vi "Bind Control Caption.vi"(4 "Ignore Past Updates? (F)":bool, 8 "error in (no error)":errorcluster, 9 "Datum Name (\"\"=Use Control Label)":string, 10 "Control Refnum":refnum<vi>, 11 "IViewable in":refnum<class "IViewable.lvclass">) -> (0 "error out":errorcluster, 3 "IViewable out":refnum<class "IViewable.lvclass">)   [LabVIEW 2018, in "MVA Framework.lvlib" / "IViewable.lvlib" / "IViewable.lvclass"]
doc: "将控制终端（控件或指示器）的标题绑定到已发布的字符串。"
uses:
  IViewable.lvclass
  mva-core/Source/IMediator/SubscriptionRequest/SubscriptionRequest.lvclass
  mva-core/Source/IObserver/IObserver Messages/Subscribe Msg/Subscribe Msg.lvclass
  <vilib>/ActorFramework/Actor/Actor.lvclass
  mva-core/Source/IMediator/ISubscriptionPolicy/ISubscriptionPolicy.lvclass
  mva-core/Source/SubscriptionPolicy/ValueChangeSubscription/ValueChangeSubscription.lvclass
  composed-transport/Source/Concrete/TerminalCaptionBinding/TerminalCaptionBinding.lvclass
  C:/Program Files (x86)/National Instruments/LabVIEW 2020/vi.lib/ActorFramework/Actor/Actor.lvclass
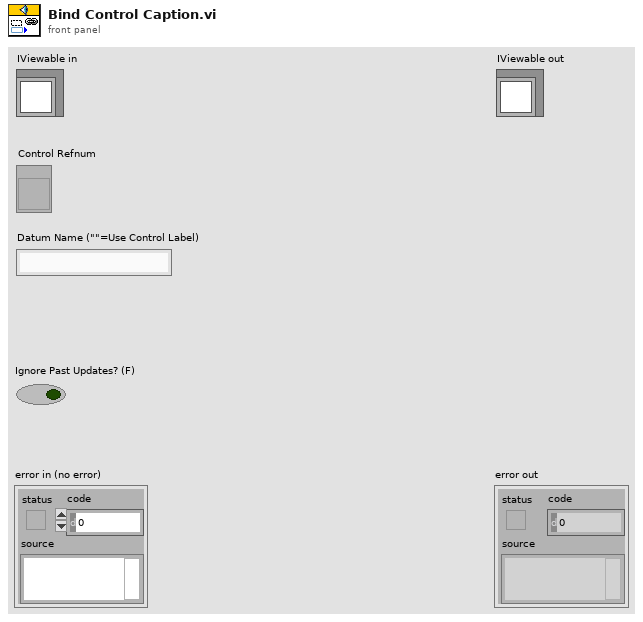
[diagram p1: front panel]
types:
  T1 = typedef "MVA Framework.lvlib/IMediator.lvlib/ISubscriptionPolicy.lvclass/ISubscriptionPolicy Reference.ctl" = refnum<data-value>
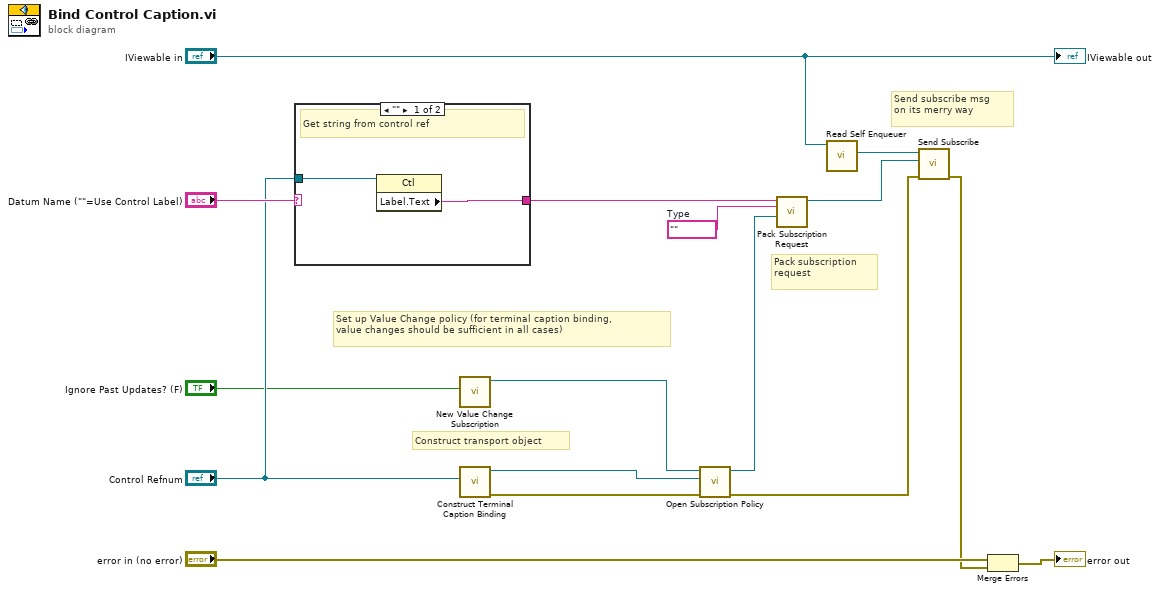
[diagram p0: block diagram]
diagram:
  w4 = ""  # Type
  # "Set up Value Change policy (for terminal caption binding,\nvalue changes should be sufficient in all cases)"
  # "Send subscribe msg\non its merry way"
  # "Pack subscription\nrequest"
  # "Construct transport object"
  n1 = case shown="\"\"" "Datum Name (\"\"=Use Control Label)" {
    selector: "Datum Name (\"\"=Use Control Label)" -> [_ w19]
    tunnel: [w17 w19] -> w10
    tunnel: "Control Refnum" -> [w18 _]
    frame "" {
      # "Get string from control ref"
      n2 = property class="Ctl"(reference=w18) -> ("Label.Text"=w17:string)  [unwired: 1 in, 2 out]
    }
    frame Default {
      # "Use string wired to input terminal"
    }
  }
  n3 = call "New Value Change Subscription.vi"("Ignore Past Updates? (F)"="Ignore Past Updates? (F)") -> ("ValueChangeSubscription Out"=w5:refnum<class "ValueChangeSubscription.lvclass">)  [unwired: 10 in]
  n4 = call "Construct Terminal Caption Binding.vi"("Ctl Refnum"="Control Refnum") -> ("error out"=w3:errorcluster, "TerminalCaptionBinding"=w8:refnum<class "TerminalCaptionBinding.lvclass">)  [unwired: 9 in]
  n5 = call "Open Subscription Policy.vi"("error in (no error)"=w3, "Transport"=w8, "SubscriptionPolicy"=w5) -> ("error out"=w2:errorcluster, "Subscription Policy"=w1:T1)  [unwired: 7 in]
  n6 = call "Pack Subscription Request.vi"("Subscription Policy"=w1, "Type"=w4, "Datum Name"=w10) -> ("SubscriptionRequest"=w7:refnum<class "SubscriptionRequest.lvclass">)  [unwired: 7 in, 1 out]
  n7 = call <vilib>:"Read Self Enqueuer.vi"("Actor"="IViewable in") -> ("Self Enqueuer"=w14:refnum<class "Message Enqueuer.lvclass">)  [unwired: 10 in]
  n8 = call "Send Subscribe.vi"("error in (no error)"=w2, "SubscriptionRequest"=w7, "Message Enqueuer"=w14) -> ("error out"=w12:errorcluster)  [unwired: 7 in, 1 out]
  n9 = Merge Errors("error in (no error)", w12) -> (→"error out":errorcluster)
  "IViewable out" <- "IViewable in"
